vi "image size control - subvi.vi"(8 "error in (no error)":errorcluster, 11 "Image Size":T1={"H Bin"=1.0, "V Bin"=1.0, "Left"=0.0, "Right"=0.0, "Top"=0.0, "Bottom"=0.0} {"V Bin" min=0.0; "H Bin" min=0.0 step=1.0}) -> (0 "error out":errorcluster)   [LabVIEW 2014]
uses:
  ctt's/Image size and binning.ctl
  Library Files - Andor and MadCity/Andorlib/atmcd32d.lvlib
panel:
  out "function return":u32
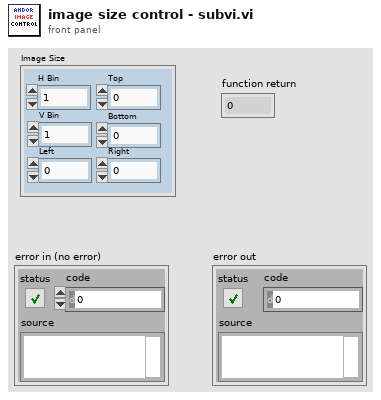
[diagram p1: front panel]
types:
  T1 = typedef "Image size and binning.ctl" = cluster{"H Bin":dbl, "V Bin":dbl, "Left":dbl, "Right":dbl, "Top":dbl, "Bottom":dbl}
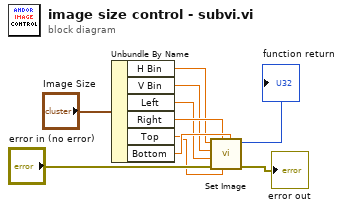
[diagram p0: block diagram]
diagram:
  n1 = Unbundle By Name("Image Size") -> ("H Bin"=w3:dbl, "V Bin"=w4:dbl, "Left"=w5:dbl, "Right"=w6:dbl, "Top"=w7:dbl, "Bottom"=w8:dbl)
  n2 = call "Set Image.vi"("vend"=w8, "vstart"=w7, "hend"=w6, "error in (no error)"="error in (no error)", "hstart"=w5, "vbin"=w4, "hbin"=w3) -> ("error out"=→"error out":errorcluster, "function return"=→"function return":u32)  [unwired: 3 in]
